vi "Write PAR_index.vi"(6 "Find all":bool=TRUE, 9 "Heater":string, 10 "EnumsPAR":string[](array[string]), 11 "Heater in":refnum<class "Heater.lvclass">) -> (1 "Not find":string[](array[string]), 2 "Find":bool, 3 "Heater out":refnum<class "Heater.lvclass">)   [LabVIEW 2019, in "Heating.lvlib" / "Heater.lvclass"]
uses:
  Heater.lvclass
  Heater.lvclass/Heater.ctl
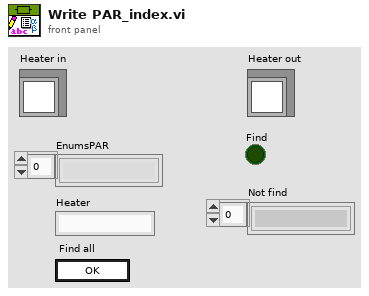
[diagram p1: front panel]
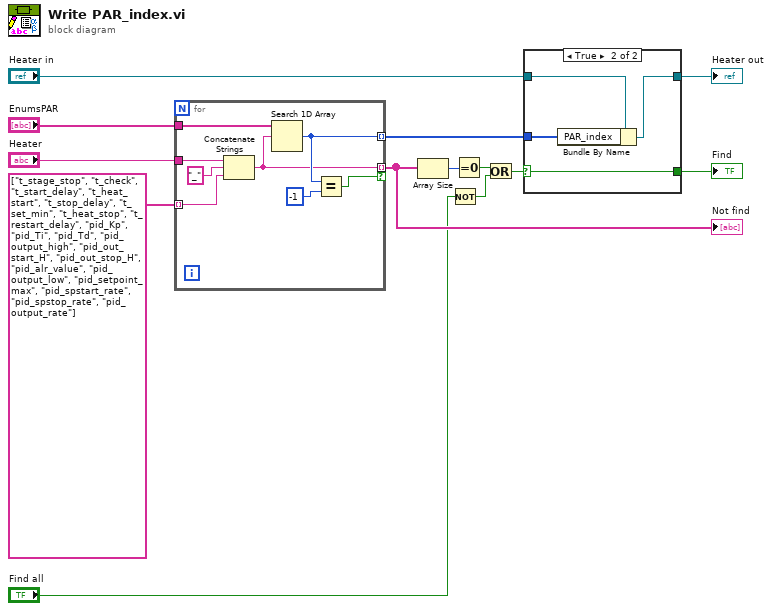
[diagram p0: block diagram]
diagram:
  n1 = for {
    tunnel: "EnumsPAR" -> [w21]
    tunnel: "Heater" -> [w20]
    tunnel: [w16] -> w12 mode=indexing
    tunnel: string[] ["t_stage_stop", "t_check", "t_start_delay", "t_heat_start", "t_stop_delay", "t_set_min", "t_heat_stop", "t_restart_delay", "pid_Kp", "pid_Ti", "pid_Td", "pid_output_high", "pid_out_start_H", "pid_out_stop_H", "pid_alr_value", "pid_output_low", "pid_setpoint_max", "pid_spstart_rate", "pid_spstop_rate", "pid_output_rate"] -> [w18] mode=indexing
    tunnel: [w15] -> w6 mode=indexing if=w14
    n2 = Concatenate Strings(w20, "_" ("string"), w18) -> (w15:string)
    n3 = Search 1D Array(1D array=w21, element=w15) -> (index of element=w16:i32)  [unwired: 1 in]
    n4 = Equal?(x=w16, y=-1 ("index of element")) -> (x = y?=w14:bool)
  }
  "Not find" <- w6
  n5 = Array Size(array=w6) -> (size(s)=w5:i32)
  n6 = Not(x="Find all") -> (.not. x?=w2:bool)
  n7 = Equal To 0?(x=w5) -> (x = 0?=w4:bool)
  n8 = Or(x=w4, y=w2) -> (x .or. y?=w3:bool)
  n9 = case shown="True" w3 {
    selector: w3 -> [_ w23]
    tunnel: [w22 w25] -> w13
    tunnel: "Heater in" -> [w22 w26]
    tunnel: w12 -> [_ w24]
    tunnel: [_ w23] -> w11
    frame False {
    }
    frame True {
      n10 = Bundle By Name(cluster=w26, "PAR_index"=w24) -> (w25:refnum<class "Heater.lvclass">)
    }
  }
  "Heater out" <- w13
  "Find" <- w11
